vi "autoconfigurator.vi"() -> ()   [LabVIEW 2012, in "MainProject.lvrbt"]
uses:
  MainProject.lvrbt
  Drivers/AutoControl3.ctl
panel:
  in  "?":path=path "C:/Users/Jeremy/Desktop/auto.conf"
  in  "?":bool
  out "?":errorcluster
  in  "?":T1[](array[typedef])
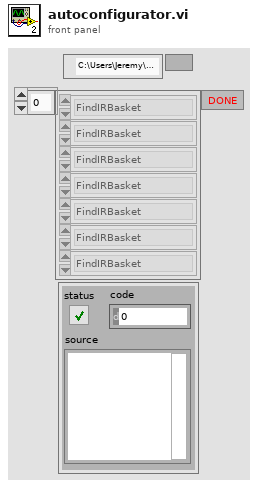
[diagram p1: front panel]
types:
  T1 = typedef "AutoControl3.ctl" = enum16{"FindIRBasket", "DropBLK", "DrvToEndOfBaskets", "DrvAroundBaskets", "AlignWithRamp", "ParkOnRamp", "Stop"}
  T2 = enum16{"open", "replace", "create", "open or create", "replace or create", "replace or create with confirmation"}
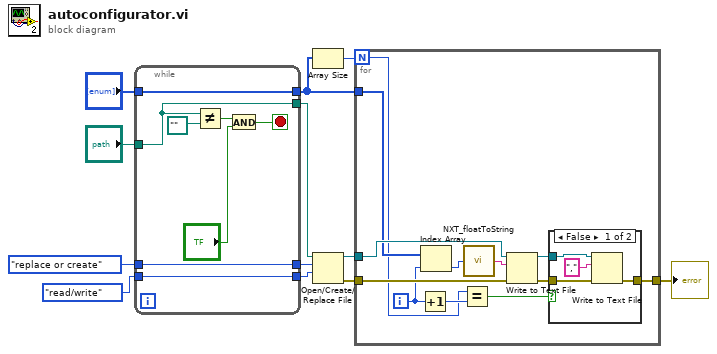
[diagram p0: block diagram]
diagram:
  n1 = while {
    tunnel: [w20] -> w3
    tunnel: "?" -> [w20]
    tunnel: "?" -> [w13]
    tunnel: [w19] -> w8
    tunnel: T2."replace or create" ("operation (0:open)") -> [w19]
    tunnel: enum16{"read/write", "read-only", "write-only"}."read/write" ("access (0:read/write)") -> [w18]
    tunnel: [w18] -> w5
    tunnel: [w13] -> w1
    stop <- w14 stop-if-true
    n2 = Not Equal?(x=w13, y=path "") -> (x != y?=w15:bool)
    n3 = And(x=w15, y="?") -> (x .and. y?=w14:bool)
  }
  n4 = Array Size(array=w3) -> (size(s)=w12:i32)
  n5 = Open/Create/Replace File(file path (use dialog)=w1, operation (0:open)=w8, access (0:read/write)=w5) -> (refnum out=w11:refnum<file>, error out=w4:errorcluster)  [unwired: 3 in, 1 out]
  n6 = for {
    N: w12 -> [w23]
    tunnel: w11 -> [w32]
    tunnel: [w29] -> w10
    tunnel: w4 -> [w25]
    tunnel: w3 -> [w24]
    i -> [w21]
    n7 = Increment(x=w21) -> (x+1=w26:i32)
    n8 = Index Array(array=w24, index=w21) -> (element=w22:T1)
    n9 = Equal?(x=w23, y=w26) -> (x = y?=w27:bool)
    n10 = call <vilib>:"NXT_floatToString.vi"("number"=w22) -> ("string"=w31:string)
    n11 = Write to Text File(file (use dialog)=w32, text=w31, error in=w25) -> (refnum out=w28:refnum<file>, error out=w30:errorcluster)  [unwired: 1 in, 1 out]
    n12 = case shown="False" w27 {
      tunnel: w30 -> [w34 w37]
      tunnel: [w33 w37] -> w29
      tunnel: w28 -> [w35 _]
      frame False {
        n13 = Write to Text File(file (use dialog)=w35, text=",", error in=w34) -> (error out=w33:errorcluster)  [unwired: 1 in, 2 out]
      }
      frame True {
      }
    }
  }
  "?" <- w10
